vi "Add Test Suite.vi"(8 "Error In (No Error)":errorcluster, 9 "Test Suite Atrributes":T1={"name"="", "tests"=-1, "failures"=-1, "errors"=-1, "time"=-1.0, "disabled"=-1, "skipped"=-1, "skips"=-1, "timestamp"=-1.0, "hostname"="", "id"="", "package"="", "assertions"=-1, "file"="", "skip"="", "log"="", "url"=""}, 10 "Teststuites Ref In":refnum<k20>, 11 "File Ref In":refnum<k20>) -> (0 "Error Out":errorcluster, 2 "Testsuite Ref":refnum<k20>, 3 "File Ref Out":refnum<k20>, 5 "Teststuites Ref Out":refnum<k20>)   [LabVIEW 2013, in "JUnit API.lvlib"]
doc: "Adds a teststuite node"
uses:
  JUnit API.lvlib
  Controls/Test Suite Attribute Values.ctl
  <vilib>/NI/Simple XML/_polymorphics/Create Tag - Child.vi
  <vilib>/NI/Simple XML/Simple XML.lvlib
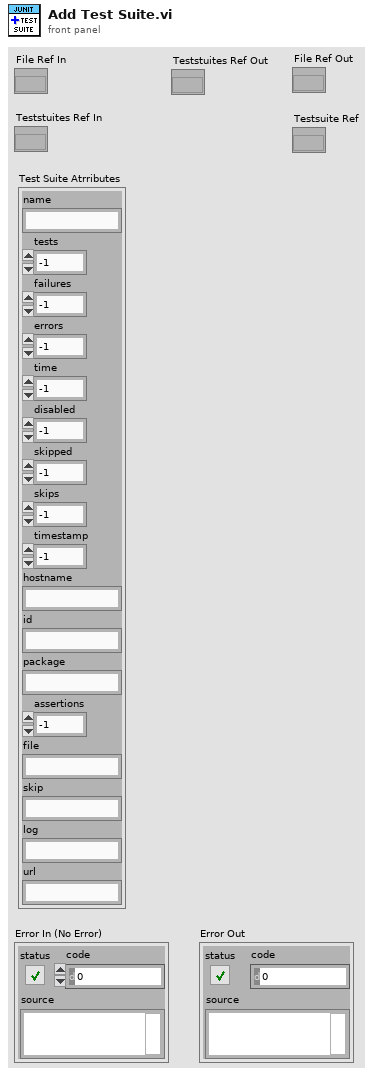
[diagram p1: front panel]
types:
  T1 = typedef "JUnit API.lvlib/Test Suite Attribute Values.ctl" = cluster{"name":string, "tests":i32, "failures":i32, "errors":i32, "time":dbl, "disabled":i32, "skipped":i32, "skips":i32, "timestamp":dbl, "hostname":string, "id":string, "package":string, "assertions":i32, "file":string, "skip":string, "log":string, "url":string}
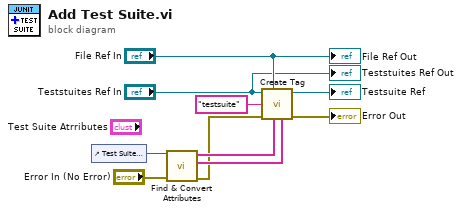
[diagram p0: block diagram]
diagram:
  n1 = control-ref of="Test Suite Atrributes"() -> (w1:refnum<vi>)
  n2 = call "Find & Convert Attributes.vi"("Error In"="Error In (No Error)", "Cluster in"=w1) -> ("Error Out"=w3:errorcluster, "Attribute Values"=w4:string[], "Attribute Names"=w5:string[])  [unwired: 7 in]
  n3 = call-poly <vilib>:"Create Tag.vi"("Attr Values"=w4, "Attr Names"=w5, "DOM Document reference"="File Ref In", "error in (no error)"=w3, "Tag Name"="testsuite", "Parent Element reference"="Teststuites Ref In") -> ("error out"=→"Error Out":errorcluster, "Child Element reference"=→"Testsuite Ref":refnum<k20>)  [unwired: 4 in]
  "File Ref Out" <- "File Ref In"
  "Teststuites Ref Out" <- "Teststuites Ref In"
